vi "Bug2 Navigation - Known Map.vi"() -> ()   [LabVIEW 2013]
doc: "This example continually replans a path from Start to Goal while following the best known path, including through obstacles if necessary.\nThe Anytime D* search algorithm is useful when the world or the robot's understanding of the world is changing. Anytime D* maintains more information than the A* search algorithm so the robot can backtrack and find a new path more easily if it discovers the original path will not work."
uses:
  <vilib>/robotics/Navigation/Anytime D Star/NI_Robotics_AnytimeDStar.lvclass
  <vilib>/robotics/Navigation/shared/WorldMap/OccupancyGridWorldMap/NI_Robotics_OccupancyGridWorldMap.lvclass
  Bug2/RVCLibrary_Bug2.lvclass
panel:
  out "y":i32
  out "x":i32
  in  "Random Obstacles?":bool
  in  "Step Through":bool
  in  "% Random Obstacles":dbl=40.0 min=0.0 max=100.0 step=1.0 format="%#_3g"
  in  "goal y":i32=35
  in  "goal x":i32=50
  out "Open List Size":i32(graph)=1665
  out "path on obstacles":dbl[][](graph)
  out "AD* Open Nodes":i32=1665 caption="size"
  out "Path Cost":dbl(graph)
  in  "Epsilon":i32=2 min=1
  out "AD* Path Cost":dbl caption="path cost"
  in  "y start":i32
  in  "x start":i32
  in  "Move Robot":i32=1 min=0
  in  "Overhaul":i32=25
  in  "step button":bool
  out "AD* Time":u32=117 caption="seconds"
  out "Compute Path Time":u32(graph)=117
  in  "stop":bool
  # "The Anytime D* search algorithm is useful when the world or the robot's understanding of the world is changing.  Anytime D* maintains more information\n than the A* search algorithm so the robot can backtrack and find a new path more easily if it discovers the original path will not work."
  # "This example continually replans a path from Start to Goal while \nfollowing the best known path, including through obstacles if necessary."
  # "Configuration"
  # "X"
  # "Y"
  # "Start"
  # "Goal"
  # "Run Mode"
  # "Run-time Control"
  # "Detection radius of robot's sensors."
  # "Number of steps the robot takes after each plan."
  # "Number of steps before AD* plans from scratch."
  # "1) Choose the Start and Goal location and the % Random Obstacles.\n2) Run the VI.\n3) Adjust the controls in the Run-time Controls section to see the \n     effect each option has on path planning\n4) Change the Run Mode to Single Step to pause after each time\n the AD* VI runs"
  # "A higher epsilon results in a faster but less optimal search."
  # "Continuous"
  # "Single Step"
  # "Robot"
  # "Obstacle"
  # "Unknown"
  # "Free"
  # "Path"
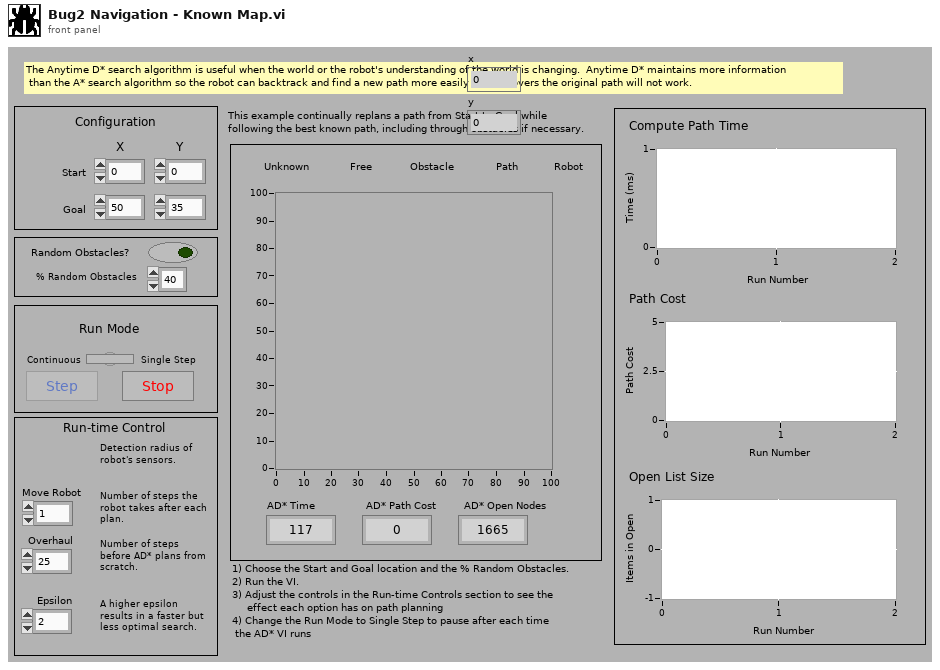
[diagram p1: front panel]
types:
  T1 = enum8{"Enabled", "Disabled", "Disabled and Grayed Out"}
  T2 = cluster{"epsilon":dbl, "run number":i32, "open list size":i32}
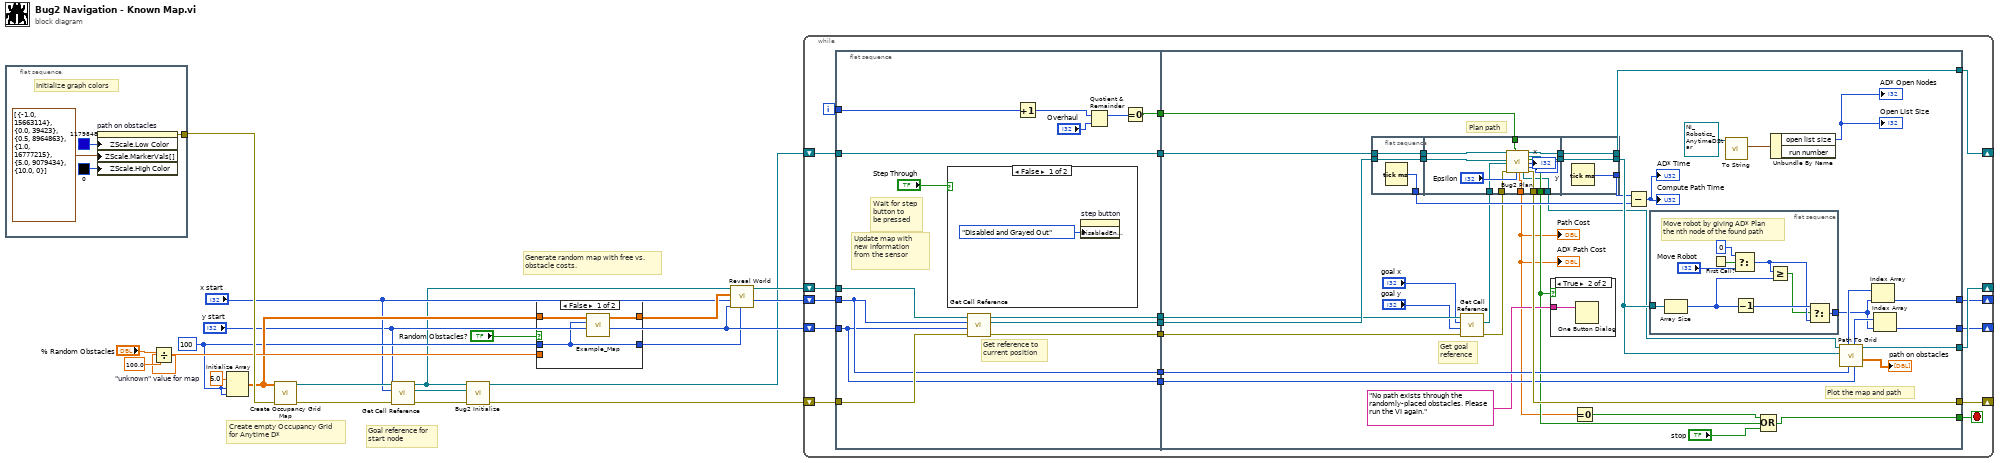
[diagram p0: block diagram]
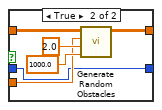
[diagram p2: hidden frame]
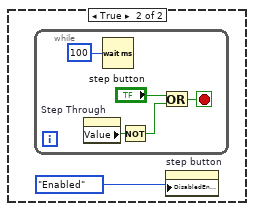
[diagram p3: hidden frame]
diagram:
  w12 = 100 ("dimension size")
  w19 = 5.0  # "unknown" value for map
  # "Goal reference for\nstart node"
  # "Generate random map with free vs.\nobstacle costs."
  # "Create empty Occupancy Grid\nfor Anytime D*"
  n1 = flat-sequence {
    tunnel: [w21] -> w16
    frame #0 {
      # "Initialize graph colors"
      n2 = property on="path on obstacles" class="IntGraph (strict)"("ZScale.Low Color"=u32 1179848, "ZScale.MarkerVals[]"=cluster{dbl, u32}[] [{-1.0, 15663114}, {0.0, 39423}, {0.5, 8964863}, {1.0, 16777215}, {5.0, 9079434}, {10.0, 0}], "ZScale.High Color"=u32 0) -> (error out=w21:errorcluster)  [unwired: 2 in, 1 out]
    }
  }
  n3 = Divide(x="% Random Obstacles", y=100.0) -> (x/y=w14:dbl)
  n4 = Initialize Array(w19, w12, w12) -> (w13:dbl[][])
  n5 = call <vilib>:"Create Occupancy Grid Map.vi"("error in (no error)"=w16, "occupancy grid"=w13) -> ("error out"=w17:errorcluster, "map reference out"=w18:refnum<data-value>)  [unwired: 8 in]
  n6 = call <vilib>:"Get Cell Reference.vi"("error in (no error)"=w17, "y"="y start", "x"="x start", "map reference in"=w18) -> ("error out"=w5:errorcluster, "cell reference"=w2:refnum<data-value>, "map reference out"=w3:refnum<data-value>)  [unwired: 4 in, 1 out]
  n7 = call "Bug2 Initialize.vi"("error in (no error)"=w5, "start reference"=w2, "map reference out"=w3) -> ("error out"=w4:errorcluster, "RVCLibrary_Bug2 out"=w1:refnum<class "RVCLibrary_Bug2.lvclass">)  [unwired: 7 in]
  n8 = case shown="False" "Random Obstacles?" {
    tunnel: w14 -> [_ w31]
    tunnel: w13 -> [w27 w30]
    tunnel: [w26 w29] -> w9
    tunnel: w12 -> [w25 w28]
    tunnel: [w25 w28] -> w6
    frame False {
      n9 = call "Example_Map.vi"("dimension size"=w25, "Array in"=w27) -> ("Array out"=w26:dbl[][])  [unwired: 9 in]
    }
    frame True {
      n10 = call "Generate Random Obstacles.vi"("obstacle cost"=1000.0, "free cost"=2.0, "chance"=w31, "cost in"=w30) -> ("cost out"=w29:dbl[][])  [unwired: 7 in]
    }
  }
  n11 = call "Reveal World.vi"("radius"=w6, "y"="y start", "x"="x start", "cost in"=w9, "map reference in"=w3) -> ("map reference in 2"=w10:refnum<data-value>)  [unwired: 5 in, 1 out]
  n12 = while {
    shift-right: [w43] -> _
    shift-left: w1 -> [w52]
    shift-right: [w50] -> _
    shift-left: w10 -> [w51]
    shift-right: [w42] -> _
    shift-left: "x start" -> [w45]
    shift-right: [w41] -> _
    shift-left: "y start" -> [w44]
    shift-right: [w36] -> _
    shift-left: w4 -> [w38]
    i -> [w40]
    stop <- w49 stop-if-true
    n13 = flat-sequence {
      tunnel: w40 -> [w60]
      tunnel: w51 -> [w54]
      tunnel: w52 -> [w66]
      tunnel: [w66] -> w48
      tunnel: [w65] -> w47
      tunnel: [w64] -> w46
      tunnel: w45 -> [w56]
      tunnel: w44 -> [w55]
      tunnel: [w59] -> w39
      tunnel: w38 -> [w58]
      tunnel: [w57] -> w37
      tunnel: [w56] -> w35
      tunnel: [w55] -> w34
      tunnel: [w79] -> w49
      tunnel: [w76] -> w43
      tunnel: [w100] -> w50
      tunnel: [w93] -> w42
      tunnel: [w92] -> w41
      tunnel: w39 -> [w98]
      tunnel: w46 -> [w97]
      tunnel: w47 -> [w91]
      tunnel: w48 -> [w108]
      tunnel: w37 -> [w88]
      tunnel: [w85] -> w36
      tunnel: w35 -> [w84]
      tunnel: w34 -> [w83]
      frame #0 {
        # "Get reference to \ncurrent position"
        # "Update map with new information\nfrom the sensor"
        # "Wait for step\nbutton to\nbe pressed"
        n14 = case shown="False" "Step Through" {
          frame False {
            n15 = property on="step button" class="Bool (strict)"("DisabledEnum"=T1."Disabled and Grayed Out" ("Disabled")) -> ()  [unwired: 2 in, 2 out]
          }
          frame True {
            n16 = while {
              stop <- w71 stop-if-true
              n17 = property on="Step Through" class="Bool (strict)"() -> ("Value"=w69:bool)  [unwired: 2 in, 2 out]
              n18 = Wait (ms)(milliseconds to wait=u32 100) -> ()  [unwired: 1 out]
              n19 = Not(x=w69) -> (.not. x?=w70:bool)
              n20 = Or(x="step button", y=w70) -> (x .or. y?=w71:bool)
            }
            n21 = property on="step button" class="Bool (strict)"("DisabledEnum"=T1."Enabled" ("Disabled")) -> ()  [unwired: 2 in, 2 out]
          }
        }
        n22 = call <vilib>:"Get Cell Reference.vi"("error in (no error)"=w58, "y"=w55, "x"=w56, "map reference in"=w54) -> ("error out"=w57:errorcluster, "cell reference"=w64:refnum<data-value>, "map reference out"=w65:refnum<data-value>)  [unwired: 4 in, 1 out]
        n23 = Increment(x=w60) -> (x+1=w62:i32)
        n24 = Quotient & Remainder(x=w62, y="Overhaul") -> (x-y*floor(x/y)=w61:i32)  [unwired: 1 out]
        n25 = Equal To 0?(x=w61) -> (x = 0?=w59:bool)
      }
      frame #1 {
        # "Plot the map and path"
        # "Get goal \nreference"
        # "Plan path"
        n26 = flat-sequence {
          tunnel: w108 -> [w123]
          tunnel: w97 -> [w124]
          tunnel: [w124] -> w107
          tunnel: [w123] -> w106
          tunnel: [w122] -> w102
          tunnel: [w134] -> w80
          tunnel: [w133] -> w78
          tunnel: w107 -> [w137]
          tunnel: w106 -> [w138]
          tunnel: [w135] -> w105
          tunnel: [w136] -> w104
          tunnel: w98 -> [w131]
          tunnel: w87 -> [w130]
          tunnel: w86 -> [w129]
          tunnel: [w128] -> w85
          tunnel: [w125] -> w74
          tunnel: [w140] -> w111
          tunnel: [w141] -> w76
          tunnel: w105 -> [w141]
          tunnel: w104 -> [w140]
          tunnel: [w139] -> w103
          frame #0 {
            n27 = Tick Count (ms)() -> (millisecond timer value=w122:u32)
          }
          frame #1 {
            n28 = call "Bug2 Plan.vi"("RVCLibrary_Bug2 in"=w138, "current reference"=w137, "new goal reference"=w130, "error in (no error)"=w129, "overhaul (F)"=w131, "epsilon"="Epsilon") -> ("path cost"=w133:dbl, "map reference out"=w125:refnum<data-value>, "RVCLibrary_Bug2 out"=w135:refnum<class "RVCLibrary_Bug2.lvclass">, "path references"=w136:refnum<data-value>[], "no valid path exists"=w134:bool, "x"=→"x":i32, "y"=→"y":i32, "error out"=w128:errorcluster)  [unwired: 6 in]
          }
          frame #2 {
            n29 = Tick Count (ms)() -> (millisecond timer value=w139:u32)
          }
        }
        n30 = call <vilib>:"Get Cell Reference.vi"("error in (no error)"=w88, "y"="goal y", "x"="goal x", "map reference in"=w91) -> ("error out"=w86:errorcluster, "cell reference"=w87:refnum<data-value>)  [unwired: 4 in, 2 out]
        n31 = case shown="True" w80 {
          tunnel: "No path exists through the randomly-placed obstacles. Please run the VI again." -> [_ w112]
          frame False {
          }
          frame True {
            n32 = One Button Dialog(message=w112) -> ()  [unwired: 1 in, 1 out]
          }
        }
        n33 = Equal To 0?(x=w78) -> (x = 0?=w77:bool)
        n34 = Subtract(x=w103, y=w102) -> (x-y=→"Compute Path Time" →"AD* Time":u32)
        n35 = flat-sequence {
          tunnel: w111 -> [w120]
          tunnel: [w113] -> w94
          frame #0 {
            # "Move robot by giving AD* Plan\nthe nth node of the found path"
            n36 = Array Size(array=w120) -> (size(s)=w117:i32)
            n37 = First Call?() -> (First Call?: T/F=w119:bool)
            n38 = Select(t=0, s=w119, f="Move Robot") -> (s? t:f=w116:i32)
            n39 = Decrement(x=w117) -> (x-1=w121:i32)
            n40 = Greater Or Equal?(x=w116, y=w117) -> (x >= y?=w115:bool)
            n41 = Select(t=w121, s=w115, f=w116) -> (s? t:f=w113:i32)
          }
        }
        n42 = call <vilib>:"To String.vi"("Anytime D* in"=refnum<class "NI_Robotics_AnytimeDStar.lvclass"> refnum) -> ("output"=w110:T2)  [unwired: 8 in, 2 out]
        n43 = Compound Arithmetic op=OR(w77, w80, "stop") -> (w79:bool)
        n44 = Unbundle By Name(w110) -> ("open list size"=→"Open List Size" →"AD* Open Nodes":i32)  [unwired: 1 out]
        n45 = call "Path To Grid.vi"("current y"=w83, "current x"=w84, "path references"=w111, "map reference in"=w74) -> ("path on obstacles"=→"path on obstacles":dbl[][], "map reference out"=w100:refnum<data-value>, "y coordinates"=w96:i32[], "x coordinates"=w95:i32[])  [unwired: 3 in, 1 out]
        n46 = Index Array(array=w95, index=w94) -> (element=w93:i32)
        n47 = Index Array(array=w96, index=w94) -> (element=w92:i32)
        "AD* Path Cost" <- w78
        "Path Cost" <- w78
      }
    }
  }
